vi "CRYAPI DOCKING.vi"(8 "sData":string, 9 "nDWinID":i32, 10 "nSWinID":i32, 11 "sAction":string) -> (0 "nData_Out":i32, 1 "sData_Out":string, 2 "tFrame_Out":T2)   [LabVIEW 2013]
uses:
  <vilib>/Utility/miscctls.llb/LVRectTypeDef.ctl
panel:
  out "bResult":bool=TRUE
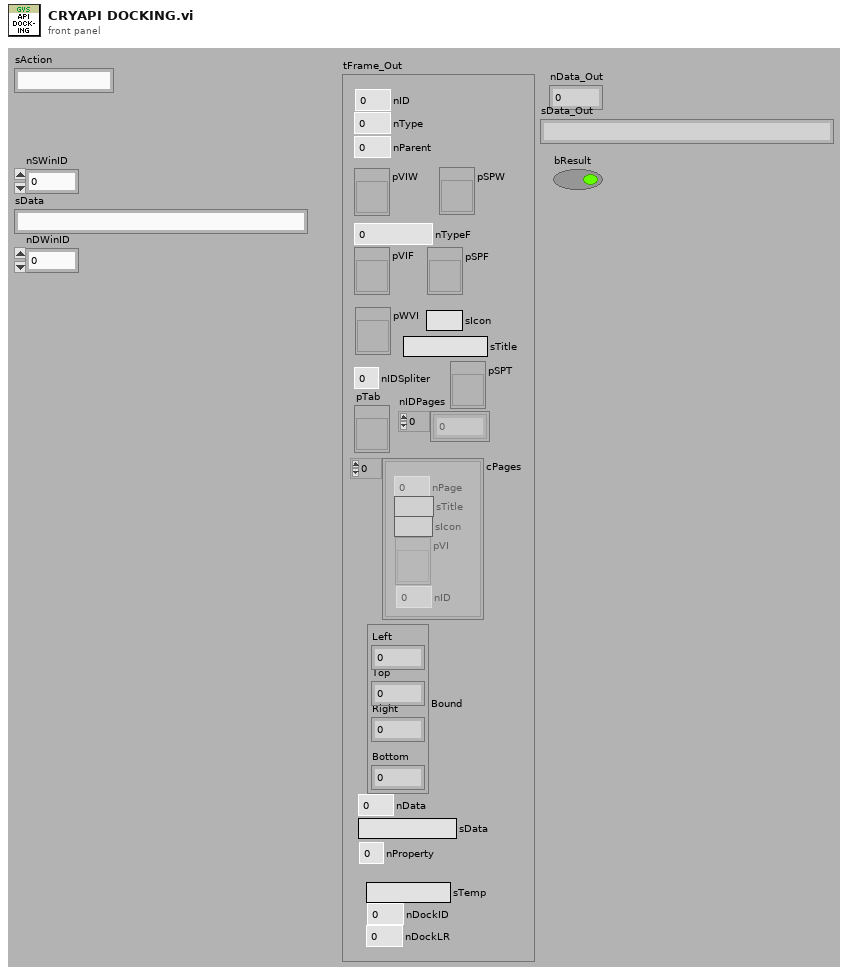
[diagram p1: front panel]
types:
  T1 = typedef "LVRectTypeDef.ctl" = cluster{"Left":i16, "Top":i16, "Right":i16, "Bottom":i16}
  T2 = cluster{"nType":i32, "nParent":i32, "pVIW":refnum<vi>, "pSPW":refnum<vi>, "nTypeF":i32, "pVIF":refnum<vi>, "pSPF":refnum<vi>, "nIDSpliter":i32, "nProperty":i32, "Bound":T1, "nID":i32, "nData":i32, "sData":string, "pWVI":refnum<vi>, "sTitle":string, "cPages":cluster{"nPage":i32, "sTitle":string, "sIcon":string, "pVI":refnum<vi>, "nID":i32}[], "pTab":refnum<vi>, "nIDPages":i32[], "pSPT":refnum<vi>, "sTemp":string, "nDockID":i32, "nDockLR":i32, "sIcon":string}
  T3 = enum16{"OK", "Yes", "YesNo", "YesNoCancel", "ReplaceAppend"}
  T4 = cluster{"nPage":i32, "sTitle":string, "sIcon":string, "pVI":refnum<vi>, "nID":i32}
  T5 = cluster{"nPage":i32, "sTitle":string, "sIcon":string, "pVI":refnum<vi>, "nID":i32}[]
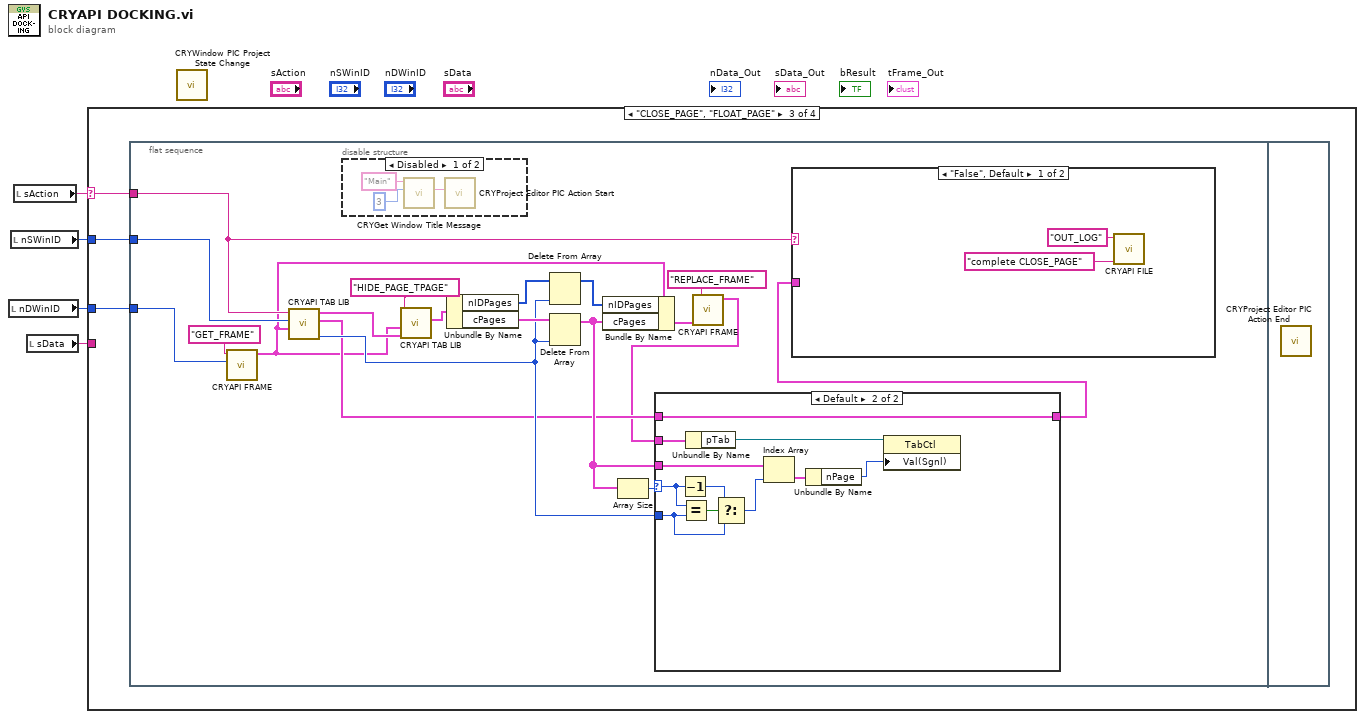
[diagram p0: block diagram]
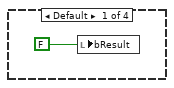
[diagram p2: hidden frame]
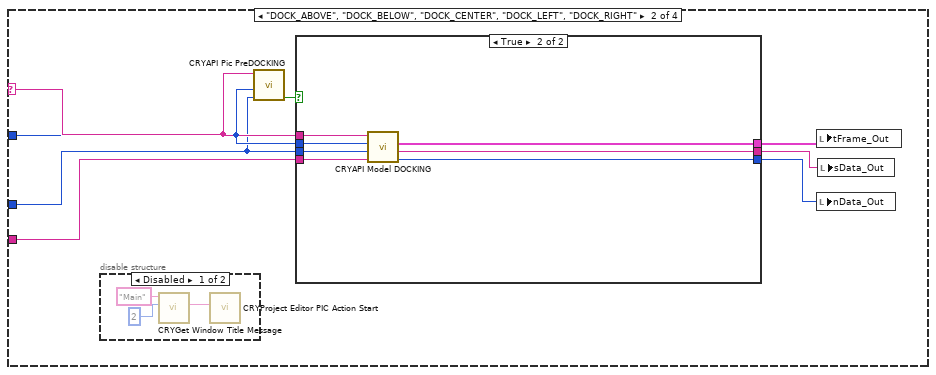
[diagram p3: hidden frame]
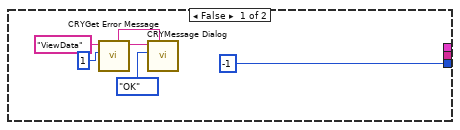
[diagram p5: hidden frame]
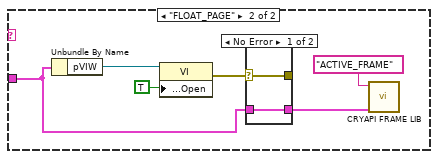
[diagram p7: hidden frame]
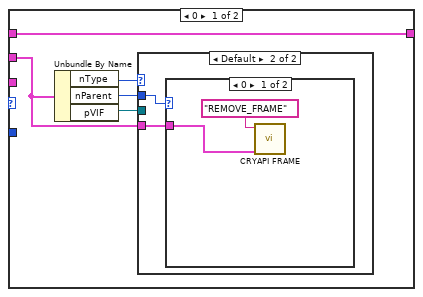
[diagram p9: hidden frame]
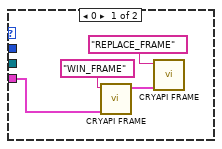
[diagram p10: hidden frame]
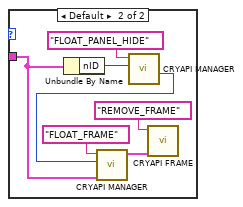
[diagram p11: hidden frame]
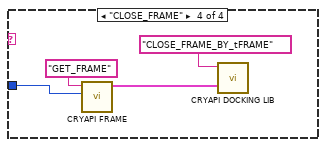
[diagram p12: hidden frame]
diagram:
  n1 = local read "nDWinID"() -> (w2:i32)
  n2 = local read "nSWinID"() -> (w3:i32)
  n3 = local read "sAction"() -> (w4:string)
  n4 = local read "sData"() -> (w1:string)
  n5 = case shown="\"CLOSE_PAGE\", \"FLOAT_PAGE\"" w4 {
    selector: w4 -> [_ w9 w31 _]
    tunnel: w3 -> [_ w7 w30 w101]
    tunnel: w2 -> [_ w6 w32 _]
    tunnel: w1 -> [_ w13 _ _]
    frame Default {
      n6 = local write "bResult"(FALSE ("bResult")) -> ()
    }
    frame "DOCK_ABOVE", "DOCK_BELOW", "DOCK_CENTER", "DOCK_LEFT", "DOCK_RIGHT" {
      n7 = disable-structure shown="Disabled" {
        frame Disabled {
          n8 = call "CRYGet Window Title Message.vi"("No"=2, "Kind"="Main") -> ("Unicode String"=w14:string)  [unwired: 4 in, 5 out]
          n9 = call "CRYProject Editor PIC Action Start.vi"("sData"=w14) -> ()  [unwired: 11 in]
        }
        frame Enabled {
        }
      }
      n10 = call "CRYAPI Pic PreDOCKING.vi"("nDWinID"=w6, "nSWinID"=w7, "sAction"=w9) -> ("bResult"=w8:bool)  [unwired: 8 in]
      n11 = case shown="True" w8 {
        tunnel: w9 -> [_ w29]
        tunnel: w7 -> [_ w28]
        tunnel: w6 -> [_ w27]
        tunnel: w13 -> [_ w26]
        tunnel: [_ w25] -> w12
        tunnel: [_ w24] -> w11
        tunnel: [-1 ("nData_Out") w23] -> w10
        frame False {
          n12 = call "CRYGet Error Message.vi"("Error No"=1, "Kind"="ViewData") -> ("Message"=w18:string, "Window Title"=w19:string)  [unwired: 4 in, 4 out]
          n13 = call "CRYMessage Dialog.vi"("Window Title"=w19, "YesNoCancel"=T3."OK", "Message Content"=w18) -> ()  [unwired: 7 in, 2 out]
        }
        frame True {
          n14 = call "CRYAPI Model DOCKING.vi"("sData"=w26, "nDWinID"=w27, "nSWinID"=w28, "sAction"=w29) -> ("nData_Out"=w23:i32, "sData_Out"=w24:string, "tFrame_Out"=w25:T2)  [unwired: 5 in]
        }
      }
      n15 = local write "tFrame_Out"(w12) -> ()
      n16 = local write "nData_Out"(w10) -> ()
      n17 = local write "sData_Out"(w11) -> ()
    }
    frame "CLOSE_PAGE", "FLOAT_PAGE" {
      n18 = flat-sequence {
        tunnel: w32 -> [w44]
        tunnel: w31 -> [w37]
        tunnel: w30 -> [w36]
        frame #0 {
          n19 = call "CRYAPI FRAME.vi"("nData"=w44, "sAction"="GET_FRAME") -> ("tFrame_Out"=w33:T2)  [unwired: 4 in, 5 out]
          n20 = call "CRYAPI TAB LIB.vi"("tFrame"=w33, "nData"=w36, "sAction"=w37) -> ("nData_Out"=w39:i32, "tFrame_Out"=w35:T2, "tPage_Out"=w47:T4)  [unwired: 1 in, 5 out]
          n21 = disable-structure shown="Disabled" {
            frame Disabled {
              n22 = call "CRYGet Window Title Message.vi"("No"=3, "Kind"="Main") -> ("Unicode String"=w52:string)  [unwired: 4 in, 5 out]
              n23 = call "CRYProject Editor PIC Action Start.vi"("sData"=w52) -> ()  [unwired: 11 in]
            }
            frame Enabled {
            }
          }
          n24 = call "CRYAPI TAB LIB.vi"("tPage"=w47, "tFrame"=w33, "sAction"="HIDE_PAGE_TPAGE") -> ("tFrame_Out"=w43:T2)  [unwired: 1 in, 7 out]
          n25 = Unbundle By Name(w43) -> ("nIDPages"=w41:i32[], "cPages"=w42:T5)
          n26 = Delete From Array(array=w41, index=w39) -> (array with subset deleted=w40:i32[])  [unwired: 1 in, 1 out]
          n27 = Delete From Array(array=w42, index=w39) -> (array with subset deleted=w51:T5)  [unwired: 1 in, 1 out]
          n28 = Bundle By Name(cluster=w33, "nIDPages"=w40, "cPages"=w51) -> (w49:T2)
          n29 = Array Size(array=w51) -> (size(s)=w50:i32)
          n30 = call "CRYAPI FRAME.vi"("tFrame"=w49, "sAction"="REPLACE_FRAME") -> ("tFrame_Out"=w34:T2)  [unwired: 4 in, 5 out]
          n31 = case shown="Default" w50 {
            selector: w50 -> [_ w95]
            tunnel: w39 -> [_ w93]
            tunnel: w34 -> [w68 w88]
            tunnel: w51 -> [_ w91]
            tunnel: w35 -> [w67 w87]
            tunnel: [w67 w87] -> w38
            frame 0 {
              n32 = Unbundle By Name(w68) -> ("nType"=w71:i32, "nParent"=w70:i32, "pVIF"=w69:refnum<vi>)
              n33 = case shown="Default" w71 {
                tunnel: w68 -> [w72 w77]
                tunnel: w70 -> [_ w76]
                tunnel: w69 -> [_ _]
                frame 0 {
                  n34 = call "CRYAPI FRAME.vi"("tFrame"=w72, "sAction"="WIN_FRAME") -> ("tFrame_Out"=w73:T2)  [unwired: 4 in, 5 out]
                  n35 = call "CRYAPI FRAME.vi"("tFrame"=w73, "sAction"="REPLACE_FRAME") -> ()  [unwired: 4 in, 6 out]
                }
                frame Default {
                  n36 = case shown="0" w76 {
                    tunnel: w77 -> [w78 w83]
                    frame 0 {
                      n37 = call "CRYAPI FRAME.vi"("tFrame"=w78, "sAction"="REMOVE_FRAME") -> ()  [unwired: 4 in, 6 out]
                    }
                    frame Default {
                      n38 = Unbundle By Name(w83) -> ("nID"=w84:i32)
                      n39 = call "CRYAPI MANAGER.vi"("nData"=w84, "sAction"="FLOAT_PANEL_HIDE") -> ("nData_Out"=w82:i32)  [unwired: 3 in, 6 out]
                      n40 = call "CRYAPI MANAGER.vi"("tFrame"=w83, "nData"=w82, "sAction"="FLOAT_FRAME") -> ("tFrame_Out"=w80:T2)  [unwired: 2 in, 6 out]
                      n41 = call "CRYAPI FRAME.vi"("tFrame"=w80, "sAction"="REMOVE_FRAME") -> ()  [unwired: 4 in, 6 out]
                    }
                  }
                }
              }
            }
            frame Default {
              n42 = Decrement(x=w95) -> (x-1=w96:i32)
              n43 = Equal?(x=w95, y=w93) -> (x = y?=w97:bool)
              n44 = Unbundle By Name(w88) -> ("pTab"=w94:refnum<vi>)
              n45 = Select(t=w96, s=w97, f=w93) -> (s? t:f=w92:i32)
              n46 = Index Array(array=w91, index=w92) -> (element=w90:T4)
              n47 = Unbundle By Name(w90) -> ("nPage"=w89:i32)
              n48 = property class="TabCtl"(reference=w94, "Val(Sgnl)"=w89) -> ()  [unwired: 1 in, 2 out]
            }
          }
          n49 = case shown="\"False\", Default" w37 {
            tunnel: w38 -> [_ w58]
            frame "False", Default {
              n50 = call "CRYAPI FILE.vi"("sData"="complete CLOSE_PAGE" ("sAction"), "sAction"="OUT_LOG") -> ()  [unwired: 8 in, 2 out]
            }
            frame "FLOAT_PAGE" {
              n51 = Unbundle By Name(w58) -> ("pVIW"=w61:refnum<vi>)
              n52 = property class="VI"(reference=w61, "Front Panel.Open"=TRUE ("Front Panel Window:Open")) -> (error out=w60:errorcluster)  [unwired: 1 in, 1 out]
              n53 = case shown="No Error" w60 {
                selector: w60 -> [w63 w65]
                tunnel: w58 -> [w64 w66]
                tunnel: [w64 w66] -> w59
                tunnel: [w63 w65] -> _
                frame No Error {
                }
                frame Error {
                }
              }
              n54 = call "CRYAPI FRAME LIB.vi"("tFrame"=w59, "sAction"="ACTIVE_FRAME") -> ()  [unwired: 4 in, 6 out]
            }
          }
        }
        frame #1 {
          n55 = call "CRYProject Editor PIC Action End.vi"() -> ()  [unwired: 12 in]
        }
      }
    }
    frame "CLOSE_FRAME" {
      n56 = call "CRYAPI FRAME.vi"("nData"=w101, "sAction"="GET_FRAME") -> ("tFrame_Out"=w98:T2)  [unwired: 4 in, 5 out]
      n57 = call "CRYAPI DOCKING LIB.vi"("tSFrame"=w98, "sAction"="CLOSE_FRAME_BY_tFRAME") -> ()  [unwired: 7 in, 3 out]
    }
  }
  n58 = call "CRYWindow PIC Project State Change.vi"() -> ()  [unwired: 12 in]
